vi "Get Outputs.vi"(8 "error in (no error)":errorcluster, 10 "Names":string[](array[string]), 11 "Node in":refnum<vi>) -> (0 "error out":errorcluster, 2 "Outputs":refnum<vi>[](array[refnum]), 3 "Node out":refnum<vi>)   [LabVIEW 2015, in "Scripting.lvlib"]
doc: "<B>bold</B>"
uses:
  Scripting.lvlib
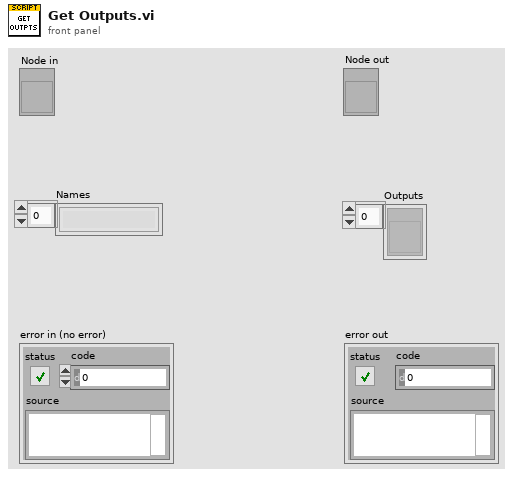
[diagram p1: front panel]
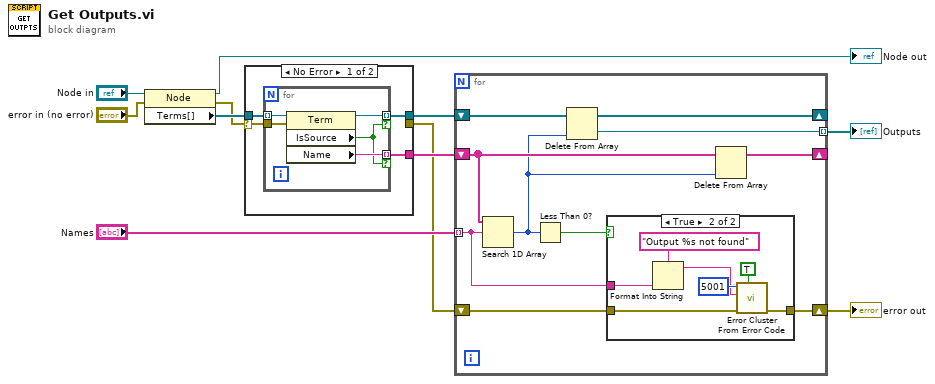
[diagram p0: block diagram]
diagram:
  n1 = property class="Node"(reference="Node in", error in="error in (no error)") -> (reference out=→"Node out":refnum<vi>, error out=w5:errorcluster, "Terms[]"=w9:refnum<vi>[])
  n2 = case shown="No Error" w5 {
    selector: w5 -> [w12 w21]
    tunnel: w9 -> [w15 _]
    tunnel: [w14 _] -> w8
    tunnel: [w13 _] -> w7
    tunnel: [_ w21] -> w4
    frame No Error {
      n3 = for {
        tunnel: w15 -> [w19] mode=indexing
        tunnel: [w20] -> w14 mode=indexing if=w16
        tunnel: [w18] -> w13 mode=indexing if=w16
        tunnel: w12 -> [w17]
        n4 = property class="Term"(reference=w19, error in=w17) -> (reference out=w20:refnum<vi>, "IsSource"=w16:bool, "Name"=w18:string)  [unwired: 1 out]
      }
    }
    frame Error {
    }
  }
  n5 = for {
    tunnel: "Names" -> [w28] mode=indexing
    shift-right: [w24] -> w3
    shift-left: w4 -> [w29]
    shift-right: [w25] -> _
    shift-left: w7 -> [w27]
    tunnel: [w23] -> w1 mode=indexing
    shift-right: [w22] -> _
    shift-left: w8 -> [w31]
    n6 = Search 1D Array(1D array=w27, element=w28) -> (index of element=w26:i32)  [unwired: 1 in]
    n7 = Less Than 0?(x=w26) -> (x < 0?=w30:bool)
    n8 = Delete From Array(array=w31, index=w26) -> (deleted portion=w23:refnum<vi>, array with subset deleted=w22:refnum<vi>[])  [unwired: 1 in]
    n9 = case shown="True" w30 {
      tunnel: w29 -> [w32 w38]
      tunnel: w28 -> [_ w36]
      tunnel: [w32 w33] -> w24
      frame False {
      }
      frame True {
        n10 = Format Into String(format string="Output %s not found", w36) -> (resulting string=w35:string)  [unwired: 2 in, 1 out]
        n11 = call <vilib>:"Error Cluster From Error Code.vi"("show call chain? (False)"=TRUE, "error in (no error)"=w38, "error message (\"\")"=w35, "error code (0)"=5001) -> ("error out"=w33:errorcluster)  [unwired: 5 in]
      }
    }
    n12 = Delete From Array(array=w27, index=w26) -> (array with subset deleted=w25:string[])  [unwired: 1 in, 1 out]
  }
  "error out" <- w3
  "Outputs" <- w1
